vi "setGamma.vi"(10 "black":u32, 11 "white":u32) -> ()   [LabVIEW 2015, in "ESLSCDLL.lvlib"]
uses:
  ESLSCDLL.lvlib
  ESLSCDLL_pro.dll
panel:
  out "error out":errorcluster
  in  "error in (no error)":errorcluster
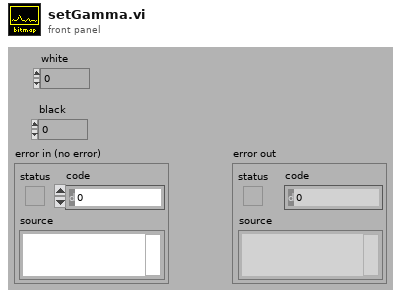
[diagram p1: front panel]
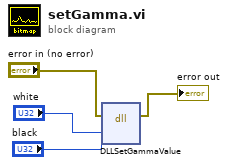
[diagram p0: block diagram]
diagram:
  n1 = dll-call lib="C:/Users/flori/Nextcloud/Dokumente/Stresing/Windows/lv64/board.vis/ESLSCDLL_pro.dll" fn="DLLSetGammaValue" ("lwlscdll.dll:DLLWriteLongS0")(error in="error in (no error)", "white"="white", "black"="black") -> (error out=→"error out":errorcluster)  [unwired: 5 in, 1 out]
